vi "Test_Buttons.vi"() -> ()   [LabVIEW 2014]
uses:
  <userlib>/UCSD Robotics Lab/Robotics-Cape/LV/libroboticscape.lvlib
panel:
  out "Timing Block":T1 {"Actual Hz" format="%#_3g"; "Dt" format="%#_4g"; "Average Hz" format="%#_4g"}
  out "Mode":bool
  out "Pause":bool
  out "State":T2(ring)
  in  "stop":bool
  # "Always stop the VI using the rectangular STOP button above, never with the round stopsign (Abort)"
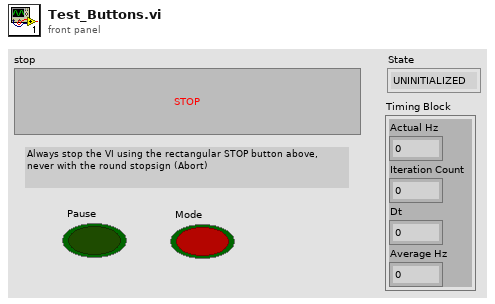
[diagram p1: front panel]
types:
  T1 = cluster{"Actual Hz":dbl, "Iteration Count":dbl, "Dt":dbl, "Average Hz":dbl}
  T2 = enum16{"UNINITIALIZED", "RUNNING", "PAUSED", "EXITING"}
  T3 = cluster{"Pause Press Event":refnum<user-event>, "Pause Release Event":refnum<user-event>, "Mode Press Event":refnum<user-event>, "Mode Release Event":refnum<user-event>}
  T4 = enum16{"UNINITIALIZED", "RUNING", "PAUSED", "EXITING"}
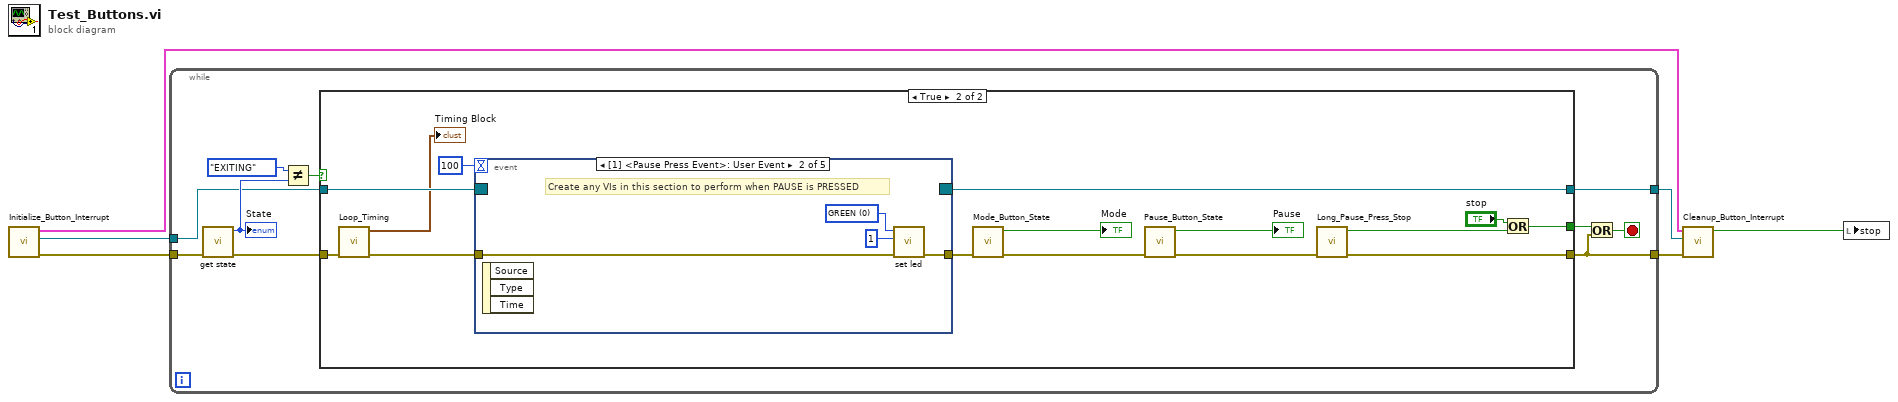
[diagram p0: block diagram]
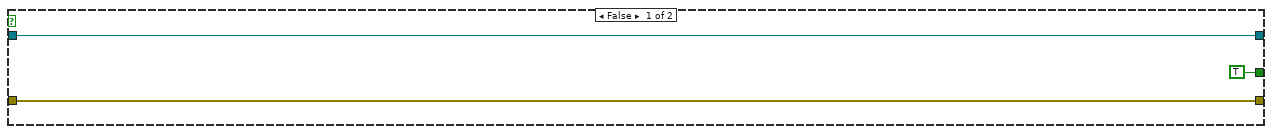
[diagram p2: hidden frame]
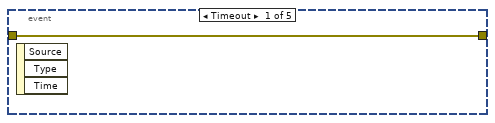
[diagram p3: hidden frame]
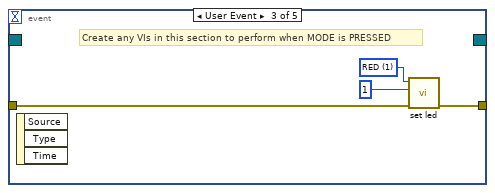
[diagram p4: hidden frame]
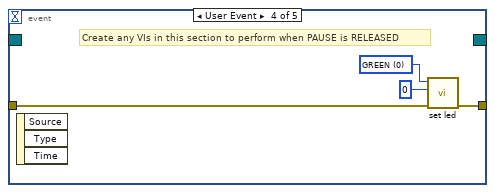
[diagram p5: hidden frame]
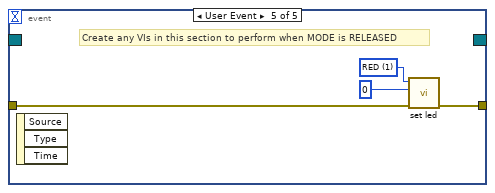
[diagram p6: hidden frame]
diagram:
  n1 = call "Initialize_Button_Interrupt.vi"() -> ("error out"=w6:errorcluster, "Event Registration Refnum 2"=w1:refnum<event-registration>, "Button Events"=w3:T3)  [unwired: 9 in]
  n2 = while {
    tunnel: w6 -> [w15]
    tunnel: [w10] -> w4
    tunnel: [w7] -> w2
    tunnel: w1 -> [w8]
    stop <- w16 stop-if-true
    n3 = call <userlib>:"get state.vi"("error in (no error)"=w15) -> ("error out"=w11:errorcluster, "function return"=w13:u32)  [unwired: 9 in]
    "State" <- w13
    n4 = Not Equal?(x=T4."EXITING" ("State 2"), y=w13) -> (x != y?=w12:bool)
    n5 = case shown="True" w12 {
      tunnel: w11 -> [w19 w27]
      tunnel: [w19 w23] -> w10
      tunnel: [TRUE ("stop") w21] -> w9
      tunnel: w8 -> [w17 w34]
      tunnel: [w17 w33] -> w7
      frame False {
      }
      frame True {
        n6 = call "Loop_Timing.vi"("error in"=w27) -> ("error out"=w26:errorcluster, "Timing Block"=→"Timing Block":T1)  [unwired: 9 in]
        n7 = event shown="[1] <Pause Press Event>: User Event" {
          selector: w34 -> [_ _ _ _ _]
          dyn-events: [_ _ _ _ _] -> w33
          timeout: 100 -> [_ _ _ _ _]
          tunnel: w26 -> [w35 w39 w43 w47 w51]
          tunnel: [w35 w38 w42 w46 w50] -> w31
          event Timeout {
            n8 = event-data() -> ()  [unwired: 1 in, 3 out]
          }
          event User Event {
            w37 = u32 0 items=["GREEN", "RED"] ("led")
            # "Create any VIs in this section to perform when PAUSE is PRESSED"
            n9 = event-data() -> ()  [unwired: 1 in, 3 out]
            n10 = call <userlib>:"set led.vi"("error in (no error)"=w39, "state"=1, "led"=w37) -> ("error out"=w38:errorcluster)  [unwired: 7 in, 1 out]
          }
          event User Event {
            w41 = u32 1 items=["GREEN", "RED"] ("led")
            # "Create any VIs in this section to perform when MODE is PRESSED"
            n11 = event-data() -> ()  [unwired: 1 in, 3 out]
            n12 = call <userlib>:"set led.vi"("error in (no error)"=w43, "state"=1, "led"=w41) -> ("error out"=w42:errorcluster)  [unwired: 7 in, 1 out]
          }
          event User Event {
            w44 = u32 0 items=["GREEN", "RED"] ("led")
            # "Create any VIs in this section to perform when PAUSE is RELEASED"
            n13 = event-data() -> ()  [unwired: 1 in, 3 out]
            n14 = call <userlib>:"set led.vi"("error in (no error)"=w47, "state"=0, "led"=w44) -> ("error out"=w46:errorcluster)  [unwired: 7 in, 1 out]
          }
          event User Event {
            w48 = u32 1 items=["GREEN", "RED"] ("led")
            # "Create any VIs in this section to perform when MODE is RELEASED"
            n15 = event-data() -> ()  [unwired: 1 in, 3 out]
            n16 = call <userlib>:"set led.vi"("error in (no error)"=w51, "state"=0, "led"=w48) -> ("error out"=w50:errorcluster)  [unwired: 7 in, 1 out]
          }
        }
        n17 = call "Mode_Button_State.vi"("error in (no error)"=w31) -> ("error out"=w30:errorcluster, "Boolean"=→"Mode":bool)  [unwired: 9 in]
        n18 = call "Pause_Button_State.vi"("error in (no error)"=w30) -> ("error out"=w24:errorcluster, "Boolean"=→"Pause":bool)  [unwired: 9 in]
        n19 = call "Long_Pause_Press_Stop.vi"("error in (no error)"=w24) -> ("error out"=w23:errorcluster, "Stop"=w20:bool)  [unwired: 9 in]
        n20 = Or(x="stop", y=w20) -> (x .or. y?=w21:bool)
      }
    }
    n21 = Or(x=w9, y=w10) -> (x .or. y?=w16:bool)
  }
  n22 = call "Cleanup_Button_Interrupt.vi"("error in (no error)"=w4, "Event Registration Refnum"=w2, "Button Events"=w3) -> ("Stop Local Variabl"=w5:bool)  [unwired: 6 in]
  n23 = local write "stop"(w5) -> ()
